vi "IPES Pressures Bk.vi"() -> ()   [LabVIEW 2010]
panel:
  out "IGC100 Prep Status":string
  out "IGC100 Main Status":string
  in  "Tab Control":T1(tab)
  out "Load Lock Backing":dbl format="%#_4e"
  out "Prep Chamber":dbl format="%#2_4e"
  out "Main Chamber":dbl format="%#_4e"
  out "Krypton":dbl format="%#_4e"
  out "Acetone":dbl format="%#_4e"
  in  "End Program":bool caption="(Safe Stop)"
  in  "Communication Interval (ms)":u32
  in  "Log Interval (s)":u32=1
  in  "Enable IGC100 Main":bool=TRUE
  in  "Enable IGC100 Prep":bool=TRUE
  out "IGC100 Prep Online":bool
  out "IGC100 Main Online":bool
  in  "IGC100 Main Port":refnum<visa-resource-name>="COM6"
  in  "IGC100 Prep Port":refnum<visa-resource-name>="COM10"
  out "IGC100 Main error":errorcluster
  out "IGC100 Prep error":errorcluster
  out "QUIT":bool
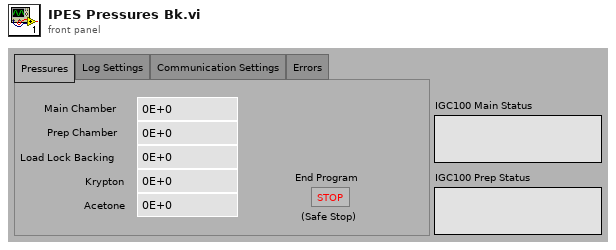
[diagram p1: front panel]
types:
  T1 = enum32{"Pressures", "Log Settings", "Communication Settings", "Errors"}
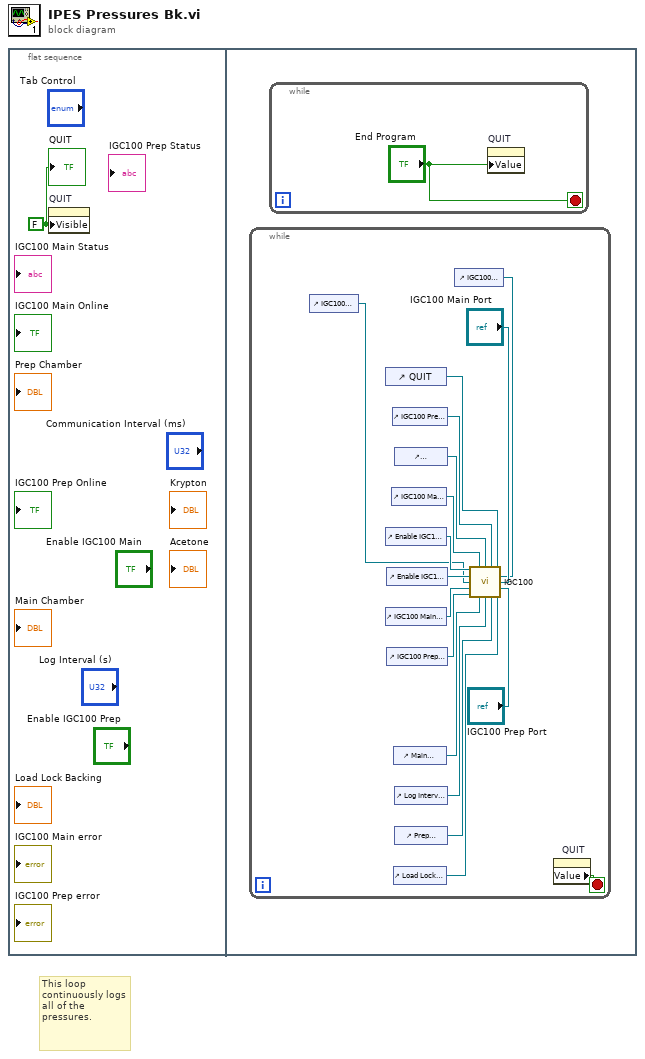
[diagram p0: block diagram]
diagram:
  # "This loop continuously logs all of the pressures."
  n1 = flat-sequence {
    frame #0 {
      w1 = FALSE ("QUIT")
      n2 = property on="QUIT" class="Bool (strict)"("Visible"=w1) -> ()  [unwired: 2 in, 2 out]
      "QUIT" <- w1
    }
    frame #1 {
      n3 = while {
        stop <- w5 stop-if-true
        n4 = control-ref of="IGC100 Prep Status"() -> (w3:refnum<vi>)
        n5 = control-ref of="QUIT"() -> (w6:refnum<vi>)
        n6 = control-ref of="Enable IGC100 Main"() -> (w11:refnum<vi>)
        n7 = control-ref of="IGC100 Main Online"() -> (w14:refnum<vi>)
        n8 = control-ref of="Enable IGC100 Prep"() -> (w12:refnum<vi>)
        n9 = control-ref of="IGC100 Prep Online"() -> (w13:refnum<vi>)
        n10 = control-ref of="IGC100 Main error"() -> (w10:refnum<vi>)
        n11 = control-ref of="IGC100 Prep error"() -> (w9:refnum<vi>)
        n12 = control-ref of="Main Chamber"() -> (w17:refnum<vi>)
        n13 = control-ref of="Load Lock Backing"() -> (w15:refnum<vi>)
        n14 = control-ref of="Communication Interval (ms)"() -> (w18:refnum<vi>)
        n15 = control-ref of="Log Interval (s)"() -> (w19:refnum<vi>)
        n16 = control-ref of="Prep Chamber"() -> (w16:refnum<vi>)
        n17 = control-ref of="IGC100 Main Status"() -> (w4:refnum<vi>)
        n18 = call "IGC100.vi"("Enable IGC100 Main"=w11, "IGC100 Main Error"=w10, "Communication Interval (s)"=w18, "IGC100 Prep Error"=w9, "QUIT"=w6, "Enable IGC100 Prep"=w12, "Main Status"=w4, "Prep Status"=w3, "IGC100 Main"="IGC100 Main Port", "IGC100 Main Online"=w14, "IGC100 Prep"="IGC100 Prep Port", "IGC100 Prep Online"=w13, "Main Chamber Pressure"=w17, "Log Interval (s)"=w19, "Prep Chamber Pressure"=w16, "Load Lock Backing Pressure"=w15) -> ()
        n19 = property on="QUIT" class="Bool (strict)"() -> ("Value"=w5:bool)  [unwired: 2 in, 2 out]
      }
      n20 = while {
        stop <- "End Program" stop-if-true
        n21 = property on="QUIT" class="Bool (strict)"("Value"="End Program") -> ()  [unwired: 2 in, 2 out]
      }
    }
  }
